vi "Set Port Speed.vi"(8 "error in":errorcluster, 10 "speed":T1, 11 "port ref":T2 format="%.0x") -> (0 "error out":errorcluster, 3 "port ref out":T2 format="%.0x")   [LabVIEW 2020, in "Ballard ARINC 429 Scripting.lvlib"]
uses:
  Ballard ARINC 429 Scripting.lvlib
  Constants.vi
  <vilib>/NI VeriStand/Custom Device API/Custom Device API.lvlib
  <vilib>/NI VeriStand/Custom Device API/Set Item Property (U16).vi
  <vilib>/NI VeriStand/Custom Device API/Custom Device Item Ref.ctl
  Shared/Transfer Speed.ctl
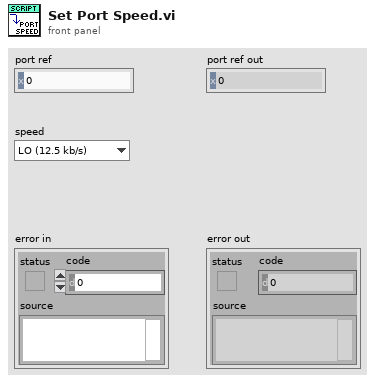
[diagram p1: front panel]
types:
  T1 = typedef "Transfer Speed.ctl" = enum16{"LO (12.5 kb/s)", "HI (100 kb/s)"}
  T2 = typedef "Custom Device API.lvlib/Custom Device Item Ref.ctl" = u64
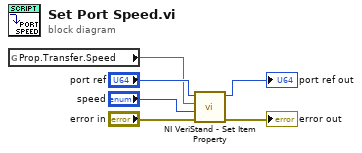
[diagram p0: block diagram]
diagram:
  n1 = global read "Constants.vi" "Prop.Transfer.Speed"() -> (w1:string)
  n2 = call-poly <vilib>:"NI VeriStand - Set Item Property.vi"("error in (no error)"="error in", "Value"="speed", "Property Name"=w1, "Item Ref in"="port ref") -> ("error out"=→"error out":errorcluster, "Item Ref out"=→"port ref out":T2)  [unwired: 5 in, 1 out]
